vi "CHECK OUT ITEM LOCATION CHECK.vi"(11 "Items Listbox":refnum<vi>) -> (3 "Change Location":bool)   [LabVIEW 2019]
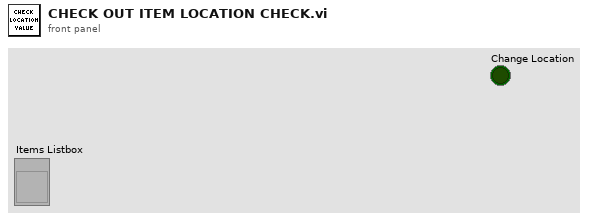
[diagram p1: front panel]
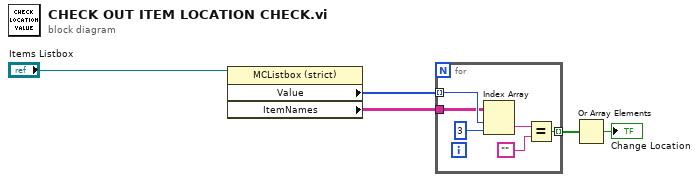
[diagram p0: block diagram]
diagram:
  n1 = property class="MCListbox (strict)"(reference="Items Listbox") -> ("Value"=w2:i32[], "ItemNames"=w1:string[][])  [unwired: 1 in, 2 out]
  n2 = for {
    tunnel: w2 -> [w8] mode=indexing
    tunnel: w1 -> [w7]
    tunnel: [w6] -> w4 mode=indexing
    n3 = Index Array(array=w7, index (row)=w8, index (col)=3 ("disabled index (col)")) -> (element=w9:string)
    n4 = Equal?(x=w9, y="") -> (x = y?=w6:bool)
  }
  n5 = Or Array Elements(Boolean array=w4) -> (logical OR=→"Change Location":bool)
